vi "ATS_Init.vi"(11 "Sampling rate":T1=2000000000 items=["400 MS/s"=400000000, "800 MS/s"=800000000, "1.2 GS/s"=1200000000, "1.6 GS/s"=1600000000, "2.0 GS/s"=2000000000]) -> (0 "error out":errorcluster, 3 "Handle":u32)   [LabVIEW 2016]
uses:
  CTL/ATS_Rate.ctl
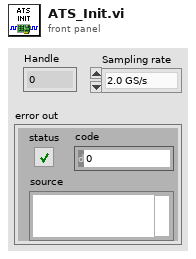
[diagram p1: front panel]
types:
  T1 = typedef "ATS_Rate.ctl" = u32
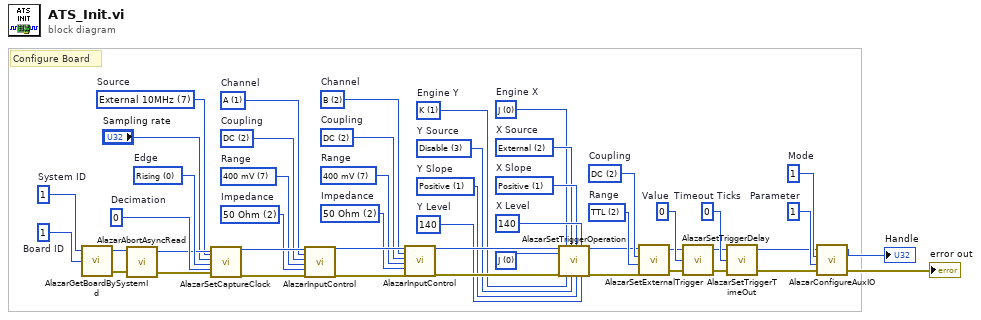
[diagram p0: block diagram]
diagram:
  w49 = u32 2 items=["TTL"=2, "2.5 V"=3]  # Range
  w19 = u32 2 items=["50 Ohm"=2]  # Impedance
  w20 = u32 7 items=["400 mV"=7]  # Range
  w18 = u32 2 items=["DC"=2]  # Coupling
  w17 = u8 2 items=["A"=1, "B"=2, "C"=4, "D"=8]  # Channel
  w40 = u32 1  # Parameter
  w41 = u32 1  # Mode
  w42 = u32 0  # Timeout Ticks
  w35 = u32 0  # Value
  w32 = u32 2 items=["AC"=1, "DC"=2]  # Coupling
  w29 = u32 140  # Y Level
  w28 = u32 1 items=["Positive"=1, "Negative"=2]  # Y Slope
  w27 = u32 3 items=["A", "B", "External", "Disable", "C", "D"]  # Y Source
  w25 = u32 140  # X Level
  w24 = u32 1 items=["Positive"=1, "Negative"=2]  # X Slope
  w23 = u32 2 items=["A", "B", "External", "Disable", "C", "D"]  # X Source
  w26 = u32 1 items=["J", "K"]  # Engine Y
  w22 = u32 0 items=["J", "K"]  # Engine X
  w21 = u32 0 items=["J", "K", "J OR K", "J AND K", "J XOR K", "J AND NOT K", "NOT J AND K"] ("Op.")
  w14 = u32 2 items=["50 Ohm"=2]  # Impedance
  w13 = u32 7 items=["400 mV"=7]  # Range
  w12 = u32 2 items=["DC"=2]  # Coupling
  w11 = u8 1 items=["A"=1, "B"=2, "C"=4, "D"=8]  # Channel
  w9 = u32 0  # Decimation
  w8 = u32 0 items=["Rising", "Falling"]  # Edge
  w6 = u32 7 items=["Internal"=1, "Fast External"=2, "Medium External"=3, "Slow External"=4, "External AC"=5, "External DC"=6, "External 10MHz"=7]  # Source
  w2 = u32 1  # Board ID
  w3 = u32 1  # System ID
  # "Configure Board"
  n1 = call "AlazarGetBoardBySystemId.vi"("Board ID"=w2, "System ID"=w3) -> ("error out"=w5:errorcluster, "Handle"=w4:u32)  [unwired: 1 in, 1 out]
  n2 = call "AlazarAbortAsyncRead.vi"("Handle"=w4, "error in (no error)"=w5) -> ("Handle"=w7:u32, "error out"=w10:errorcluster)  [unwired: 1 out]
  n3 = call "AlazarSetCaptureClock.vi"("Handle"=w7, "Source"=w6, "Sample Rate"="Sampling rate", "Edge"=w8, "Decimation"=w9, "error in (no error)"=w10) -> ("Handle"=w15:u32, "error out"=w16:errorcluster)  [unwired: 11 in, 1 out]
  n4 = call "AlazarInputControl.vi"("Handle"=w15, "Channel"=w11, "Coupling"=w12, "Range"=w13, "Impedance"=w14, "error in (no error)"=w16) -> ("Handle"=w46:u32, "error out"=w43:errorcluster)  [unwired: 11 in, 1 out]
  n5 = call "AlazarInputControl.vi"("Handle"=w46, "Channel"=w17, "Coupling"=w18, "Range"=w20, "Impedance"=w19, "error in (no error)"=w43) -> ("Handle"=w45:u32, "error out"=w44:errorcluster)  [unwired: 11 in, 1 out]
  n6 = call "AlazarSetTriggerOperation.vi"("Handle"=w45, "Operation"=w21, "error in (no error)"=w44, "Engine X"=w22, "Engine Y"=w26, "X Source"=w23, "Y Source"=w27, "X Slope"=w24, "Y Slope"=w28, "X Level"=w25, "Y Level"=w29) -> ("Handle"=w30:u32, "error out"=w31:errorcluster)  [unwired: 6 in, 1 out]
  n7 = call "AlazarSetExternalTrigger.vi"("error in (no error)"=w31, "Range"=w49, "Coupling"=w32, "Handle"=w30) -> ("error out"=w34:errorcluster, "Handle"=w33:u32)  [unwired: 1 out]
  n8 = call "AlazarSetTriggerDelay.vi"("error in (no error)"=w34, "Value"=w35, "Handle"=w33) -> ("error out"=w37:errorcluster, "Handle"=w36:u32)  [unwired: 1 out]
  n9 = call "AlazarSetTriggerTimeOut.vi"("error in (no error)"=w37, "Timeout Ticks"=w42, "Handle"=w36) -> ("error out"=w39:errorcluster, "Handle"=w38:u32)  [unwired: 1 out]
  n10 = call "AlazarConfigureAuxIO.vi"("error in (no error)"=w39, "Parameter"=w40, "Mode"=w41, "Handle"=w38) -> ("error out"=→"error out":errorcluster, "Handle"=→"Handle":u32)  [unwired: 1 out]
